vi "DownloadSoftware_EV3.vi"() -> ()   [LabVIEW 2012]
uses:
  SubVIs/LVPresent_Globals.vi
  <vilib>/Platform/browser.llb/Open URL in Default Browser (string).vi
panel:
  in  "For Windows":bool caption="Click here!"
  in  "For Mac":bool caption="Click here!"
  in  "Click here!":bool
  # "Downloading the Software\n\nFirst, make sure that you have LabVIEW 2012 on your computer.  Then, follow the two steps below to download LabVIEW 2012 SP1 Module for LEGO MINDSTORMS. Beware that there are different versions for Windows and Mac operating systems for both steps."
  # "Step 1:"
  # "Step 2:"
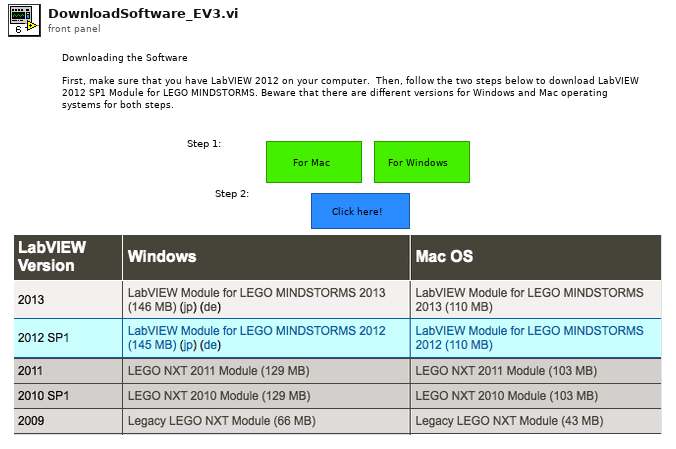
[diagram p1: front panel]
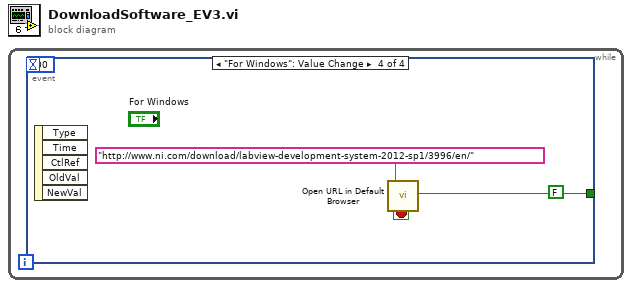
[diagram p0: block diagram]
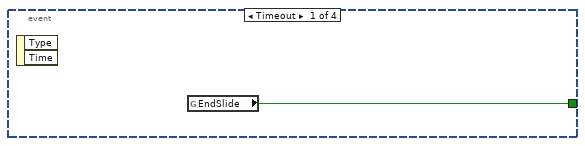
[diagram p2: hidden frame]
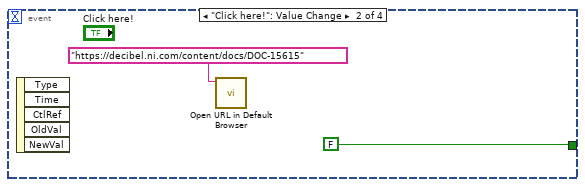
[diagram p3: hidden frame]
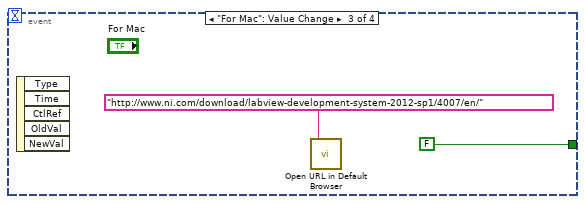
[diagram p4: hidden frame]
diagram:
  n1 = while {
    stop <- w2 stop-if-true
    n2 = event shown="[3] \"For Windows\": Value Change" {
      selector: _ -> [_ _ _ _]
      dyn-events: _ -> [_ _ _ _]
      timeout: 500 -> [_ _ _ _]
      tunnel: [w3 FALSE FALSE FALSE] -> w2
      event Timeout {
        n3 = event-data() -> ()  [unwired: 1 in, 2 out]
        n4 = global read "LVPresent_Globals.vi" "EndSlide"() -> (w3:bool)
      }
      event "Click here!": Value Change {
        n5 = event-data() -> ()  [unwired: 1 in, 5 out]
        n6 = call-poly <vilib>:"Open URL in Default Browser.vi"("URL"="https://decibel.ni.com/content/docs/DOC-15615") -> ()  [unwired: 5 in, 2 out]
      }
      event "For Mac": Value Change {
        n7 = event-data() -> ()  [unwired: 1 in, 5 out]
        n8 = call-poly <vilib>:"Open URL in Default Browser.vi"("URL"="http://www.ni.com/download/labview-development-system-2012-sp1/4007/en/") -> ()  [unwired: 5 in, 2 out]
      }
      event "For Windows": Value Change {
        n9 = event-data() -> ()  [unwired: 1 in, 5 out]
        n10 = call-poly <vilib>:"Open URL in Default Browser.vi"("URL"="http://www.ni.com/download/labview-development-system-2012-sp1/3996/en/") -> ()  [unwired: 5 in, 2 out]
      }
    }
  }
